vi "示例 7.vi"() -> ()   [LabVIEW 2021]
panel:
  out "XY Graph":cluster{"Y":dbl[], "Y":dbl[]}[](graph)
  in  "stop":bool
  in  "d":dbl
  in  "r":dbl
  in  "R":dbl
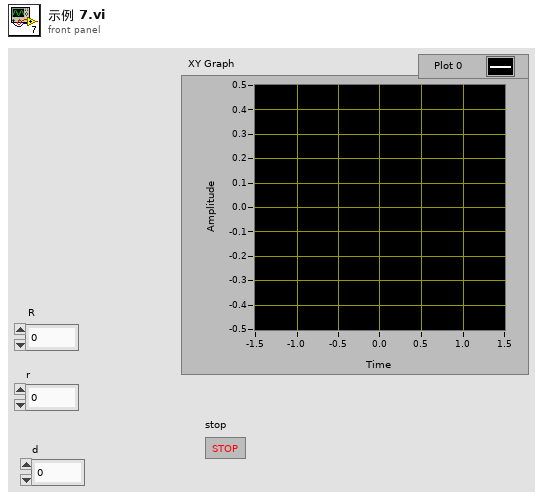
[diagram p1: front panel]
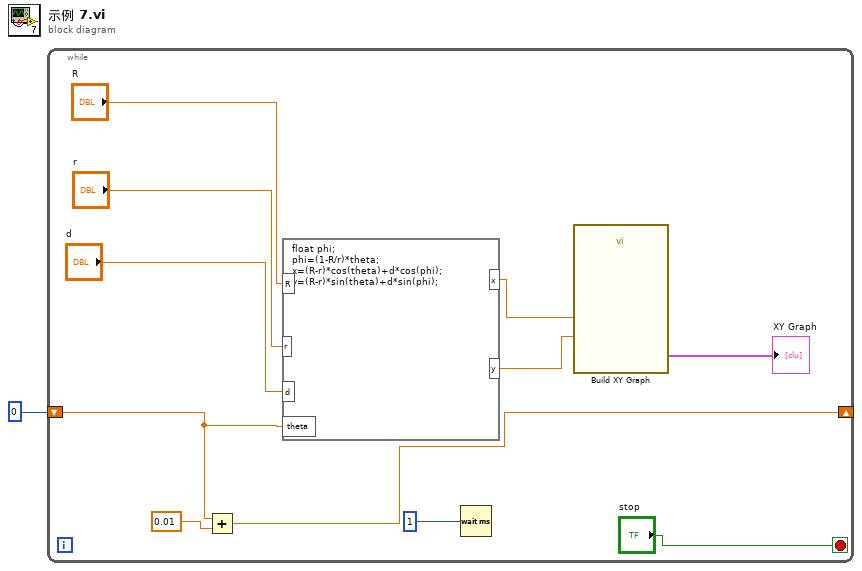
[diagram p0: block diagram]
diagram:
  n1 = while {
    shift-right: [w2] -> _
    shift-left: 0 -> [w8]
    stop <- "stop" stop-if-true
    n2 = Add(x=w8, y=0.01) -> (x+y=w2:dbl)
    n3 = formula code="float phi;\nphi=(1-R/r)*theta;\nx=(R-r)*cos(theta)+d*cos(phi);\ny=(R-r)*sin(theta)+d*sin(phi);"("R"="R", "r"="r", "d"="d", "theta"=w8) -> ("x"=w4:dbl, "y"=w3:dbl)
    n4 = Wait (ms)(milliseconds to wait=1) -> ()  [unwired: 1 out]
    n5 = call "Build XY Graph"("Y Input"=w3, "X Input"=w4) -> ("XY Graph"=→"XY Graph":cluster{"X":dbl[], "Y":dbl[]}[])  [unwired: 8 in, 1 out]
  }
